vi "dvp Vi Get Awb Operation.vi"(10 "pAwbOperation":u32(ring) items=["AWB_OP_OFF", "AWB_OP_ONCE", "AWB_OP_CONTINUOUS"], 11 "handle":u32) -> (2 "pAwbOperation out":u32(ring) items=["AWB_OP_OFF", "AWB_OP_ONCE", "AWB_OP_CONTINUOUS"], 3 "function return":u32(ring))   [LabVIEW 2018, in "LabViewDVPCamera.lvlib"]
doc: "LabviewDvp2Api dvpStatus dvpViGetAwbOperation(dvpHandle handle, dvpAwbOperation *pAwbOperation);"
uses:
  LabViewDVPCamera.lvlib
  LabViewDVPCamera/LabViewDVPCamera.dll
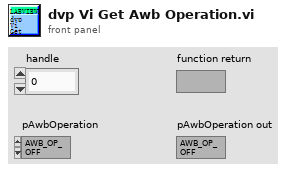
[diagram p1: front panel]
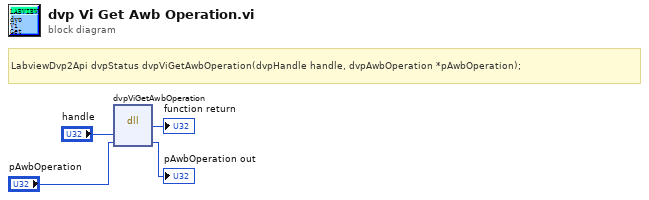
[diagram p0: block diagram]
diagram:
  # "LabviewDvp2Api dvpStatus dvpViGetAwbOperation(dvpHandle handle, dvpAwbOperation *pAwbOperation);"
  n1 = dll-call lib="C:/Program Files (x86)/DVP2 Labview cn 64/Sample/LabViewDVPCamera/LabViewDVPCamera.*" fn="dvpViGetAwbOperation"("handle"="handle", "pAwbOperation"="pAwbOperation") -> (→"function return":u32, "pAwbOperation"=→"pAwbOperation out":u32)  [unwired: 4 in, 2 out]
